vi "Disconnect.vi"(8 "Error In":errorcluster, 10 "Description":string="Normal Shutdown", 11 "Session In":refnum<class "Session.lvclass">) -> (0 "Error Out":errorcluster, 3 "Sesssion Out":refnum<class "Session.lvclass">)   [LabVIEW 2018, in "Toolkit.lvlib" / "Session.lvclass"]
uses:
  Session.lvclass
  Session.lvclass/Session.ctl
  SSH/SSH.lvclass/SSH.ctl
  Toolkit.lvlib
  SSH/SSH.lvclass
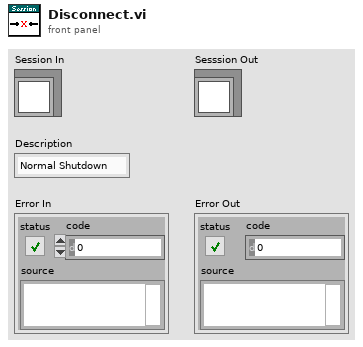
[diagram p1: front panel]
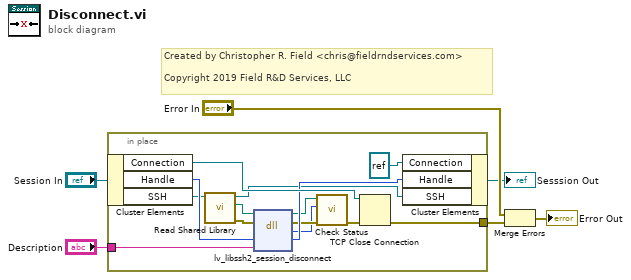
[diagram p0: block diagram]
diagram:
  # "Created by Christopher R. Field <chris@fieldrndservices.com>\n\nCopyright 2019 Field R&D Services, LLC"
  n1 = in-place {
    in-place-border: "Description" -> [w18]
    in-place-border: [w16] -> w1
    n2 = in-place-cluster #1("Session In") -> ("Connection"=w20:refnum<k5>, "Handle"=w15:u64, "SSH"=w10:refnum<class "SSH.lvclass">)
    n3 = call "Read Shared Library.vi"("SSH In"=w10) -> ("Error Out"=w8:errorcluster, "lv-libssh2 Shared Library"=w7:path, "SSH Out"=w9:refnum<class "SSH.lvclass">)  [unwired: 8 in]
    n4 = dll-call lib="D:/Users/cfield/Code/Field R&D Services/SSH/LV-LIBSSH2/LabVIEW/trunk/src/Toolkit/Support/lv-libssh2.*" fn="lv_libssh2_session_disconnect"(path in=w7, error in=w8, "session"=w15, "description"=w18) -> (path out=w13:path, error out=w14:errorcluster, "result"=w11:i32, "session"=w17:u64)  [unwired: 2 in]
    n5 = call "Check Status.vi"("Error In"=w14, "Status"=w11, "lv-libssh2 Shared Library In"=w13) -> ("Error Out"=w12:errorcluster)  [unwired: 7 in, 1 out]
    n6 = TCP Close Connection(connection ID=w20, error in (no error)=w12) -> (error out=w16:errorcluster)  [unwired: 1 in, 1 out]
    n7 = in-place-cluster #1("Connection"=refnum<k5> refnum, "Handle"=w17, "SSH"=w9) -> (→"Sesssion Out":refnum<class "Session.lvclass">)
  }
  n8 = Merge Errors("Error In", w1) -> (→"Error Out":errorcluster)
